vi "Check for duplicates in spreadsheet or csv file with list of field numbers.vi"(7 "2D data table":string[][](array[string]), 8 "error in (no error)":errorcluster, 9 "Use 2D data not file (F)?":bool, 10 "Fields table":u32[](array[numeric]), 11 "file path (dialog if empty)":path) -> (0 "error out":errorcluster, 3 "Duplicates?":bool)   [LabVIEW 2013]
uses:
  <vilib>/Utility/file.llb/Read From Spreadsheet File (string).vi
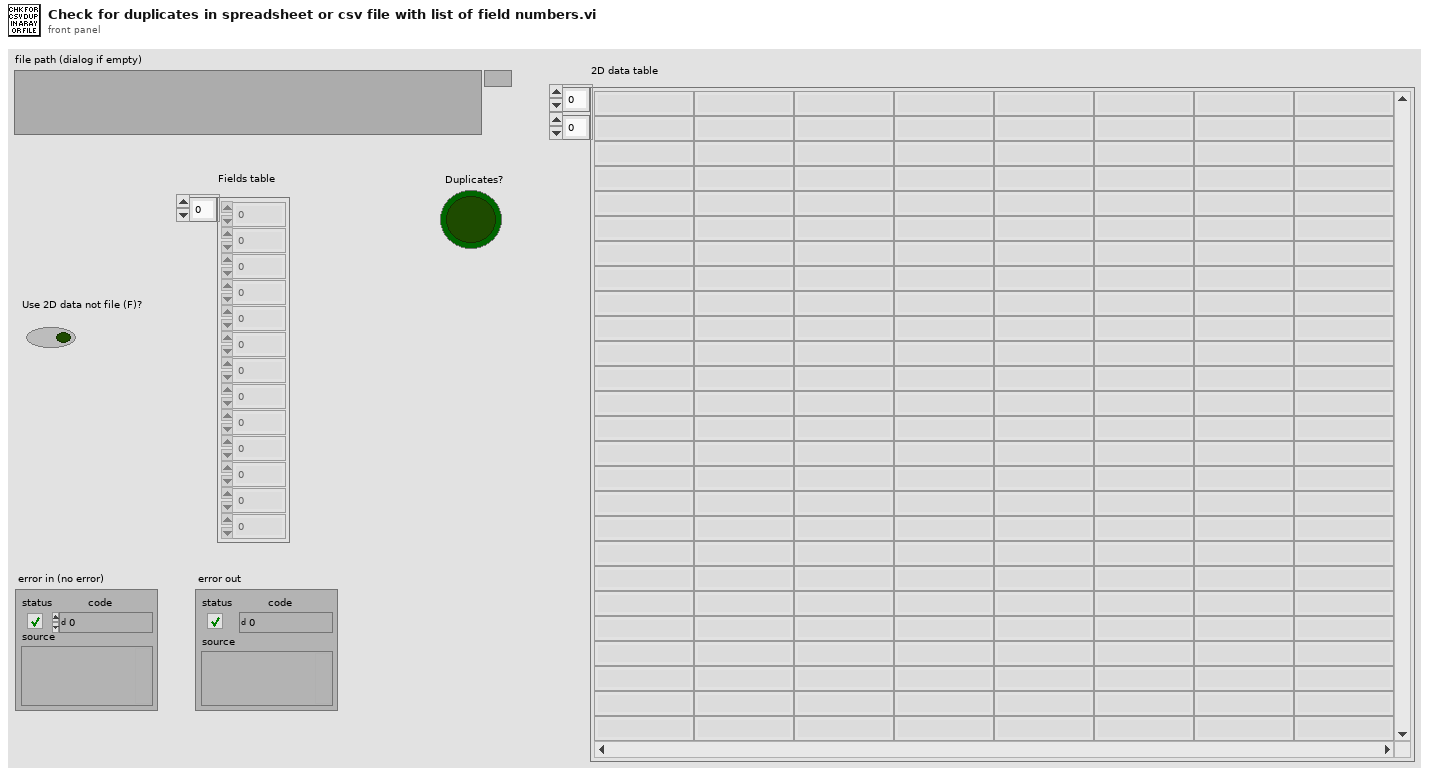
[diagram p1: front panel]
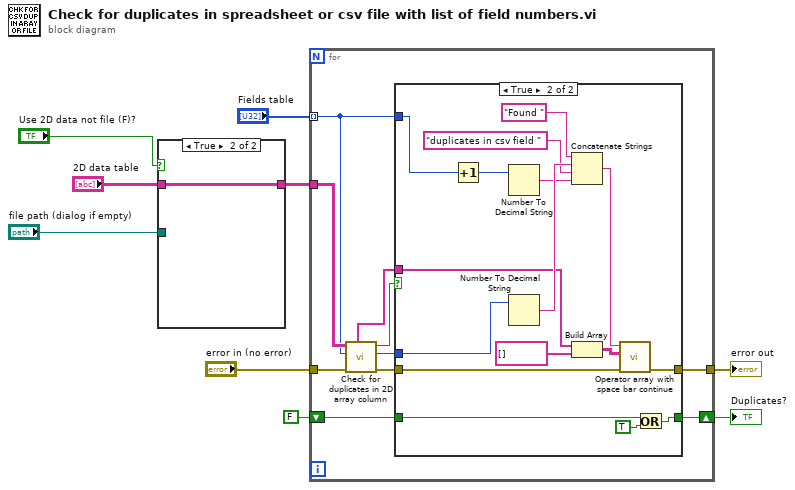
[diagram p0: block diagram]
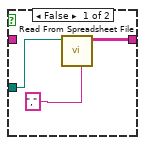
[diagram p2: hidden frame]
diagram:
  n1 = case shown="True" "Use 2D data not file (F)?" {
    tunnel: [w11 w13] -> w8
    tunnel: "file path (dialog if empty)" -> [w10 _]
    tunnel: "2D data table" -> [_ w13]
    frame False {
      n2 = call-poly <vilib>:"Read From Spreadsheet File.vi"("delimiter (\\t)"="," ("delimiter (\\t)"), "file path (dialog if empty)"=w10) -> ("all rows"=w11:string[][])  [unwired: 5 in, 4 out]
    }
    frame True {
    }
  }
  n3 = for {
    tunnel: "Fields table" -> [w19] mode=indexing
    tunnel: w8 -> [w23]
    tunnel: "error in (no error)" -> [w22]
    tunnel: [w16] -> w6
    shift-right: [w14] -> w4
    shift-left: FALSE -> [w15]
    n4 = call "Check for duplicates in 2D array column.vi"("error in (no error)"=w22, "CSV field (0-N)"=w19, "Array"=w23) -> ("error out"=w17:errorcluster, "Duplicates Count"=w20:i32, "Got duplicates?"=w21:bool, "Duplicate data"=w18:string[])  [unwired: 2 in, 3 out]
    n5 = case shown="True" w21 {
      tunnel: w20 -> [_ w40]
      tunnel: w19 -> [_ w36]
      tunnel: w18 -> [_ w33]
      tunnel: w17 -> [w25 w30]
      tunnel: [w25 w29] -> w16
      tunnel: w15 -> [w24 w28]
      tunnel: [w24 w26] -> w14
      frame False {
      }
      frame True {
        n6 = Increment(x=w36) -> (x+1=w35:u32)
        n7 = Number To Decimal String(number=w35) -> (decimal integer string=w37:string)  [unwired: 1 in]
        n8 = Number To Decimal String(number=w40) -> (decimal integer string=w39:string)  [unwired: 1 in]
        n9 = Concatenate Strings("Found " ("string"), w39, "duplicates in csv field " ("string"), w37) -> (w34:string)
        n10 = Build Array(w33, string[] [] ("element")) -> (w31:string[][])
        n11 = call "Operator array with space bar continue.vi"("error in (no error)"=w30, "Array"=w31, "Message"=w34) -> ("error out"=w29:errorcluster)  [unwired: 7 in, 1 out]
        n12 = Or(x=w28, y=TRUE) -> (x .or. y?=w26:bool)
      }
    }
  }
  "error out" <- w6
  "Duplicates?" <- w4
